vi "Query LAN Trigger Connection Status.vi"(8 "error in (no error)":errorcluster, 10 "Trigger Number (1)":i32=1, 11 "VISA resource name":refnum<visa-resource-name>) -> (0 "error out":errorcluster, 2 "LAN Connected":bool, 3 "VISA resource name out":refnum<visa-resource-name>)   [LabVIEW 2017, in "Keithley 2600 Series.lvlib"]
doc: "Returns the LAN event connection state."
uses:
  <instrlib>/Keithley 2600 Series/Keithley 2600 Series.lvlib
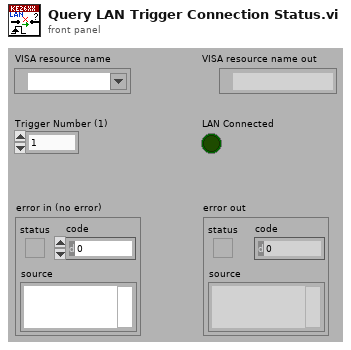
[diagram p1: front panel]
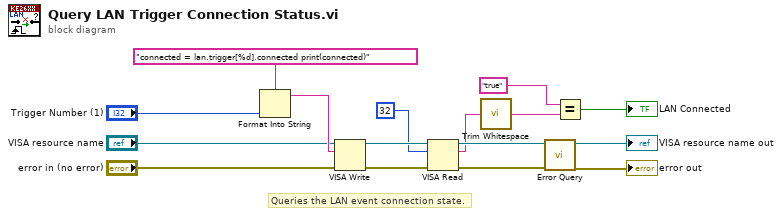
[diagram p0: block diagram]
diagram:
  # "Queries the LAN event connection state."
  n1 = Format Into String(format string="connected = lan.trigger[%d].connected print(connected)", "Trigger Number (1)") -> (resulting string=w14:string)  [unwired: 2 in, 1 out]
  n2 = VISA Write(VISA resource name="VISA resource name", write buffer=w14, error in (no error)="error in (no error)") -> (VISA resource name out=w7:refnum<visa-resource-name>, error out=w6:errorcluster)  [unwired: 1 out]
  n3 = VISA Read(VISA resource name=w7, byte count=u32 32, error in (no error)=w6) -> (VISA resource name out=w8:refnum<visa-resource-name>, read buffer=w3:string, error out=w9:errorcluster)  [unwired: 1 out]
  n4 = call <vilib>:"Trim Whitespace.vi"("string"=w3) -> ("trimmed string"=w2:string)  [unwired: 1 in]
  n5 = call <instrlib>:"Error Query.vi"("error in (no error)"=w9, "VISA resource name"=w8) -> ("error out"=→"error out":errorcluster, "VISA resource name out"=→"VISA resource name out":refnum<visa-resource-name>)  [unwired: 6 in, 2 out]
  n6 = Equal?(x="true", y=w2) -> (x = y?=→"LAN Connected":bool)
